vi "size_to_temperature.vi"(9 "Drop Time":dbl, 10 "sigma":dbl, 11 "Pixel Size":dbl) -> (2 "Temperature (K)":dbl)   [LabVIEW 2016]
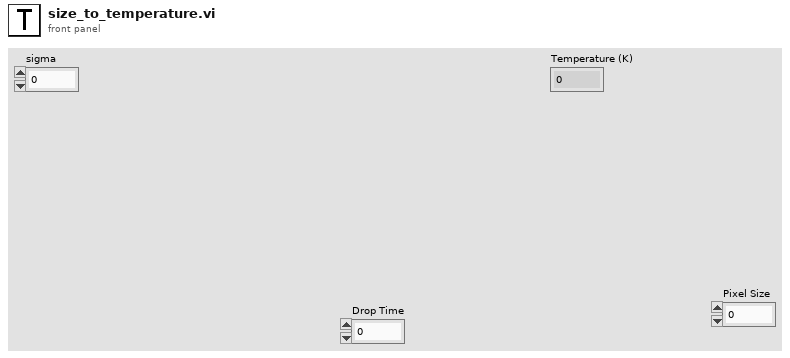
[diagram p1: front panel]
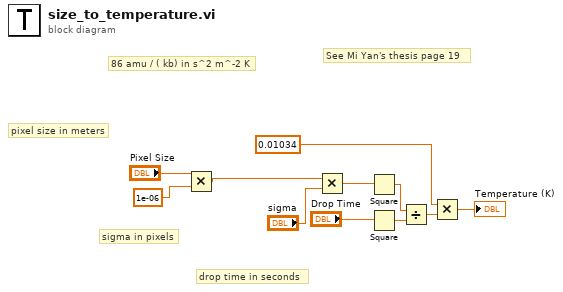
[diagram p0: block diagram]
diagram:
  # "See Mi Yan's thesis page 19"
  # "drop time in seconds"
  # "sigma in pixels"
  # "pixel size in meters"
  # "86 amu / ( kb) in s^2 m^-2 K"
  n1 = Multiply(x="Pixel Size", y=1e-06) -> (x*y=w1:dbl)
  n2 = Multiply(x=w1, y="sigma") -> (x*y=w11:dbl)
  n3 = Square(x=w11) -> (x^2=w8:dbl)
  n4 = Square(x="Drop Time") -> (x^2=w9:dbl)
  n5 = Divide(x=w8, y=w9) -> (x/y=w7:dbl)
  n6 = Multiply(x=0.01034, y=w7) -> (x*y=→"Temperature (K)":dbl)
